vi "util-path.vi"(6 "Create Folders?(F)":bool, 8 "error in":errorcluster, 10 "Selected Folder (PROCS)":T1, 11 "append path (ie. folder\\filename.*)":string) -> (0 "error out":errorcluster, 1 "SelectedPath Filenames":string[](array[string]), 2 "SelectedPath":path, 3 "AppPath":path, 4 ".extension (.prc)":string)   [LabVIEW 2024]
uses:
  controls/typePathSelector.ctl
panel:
  # "path to file:  folder1\\...\\filename.*"
  # "build path example:\n\nAppend to may be a path to folder (123\\456) or a path to file (123\\456.*)\n\nif specific folder is selected (Procedures, templates, logs etc.) the code tries \nto add a file extansion by replacing *. in the provided path (Append To)\n\nif there is no filename (hence no .* at the end) the path in Append To considered \npath to folder.\n\nAppend To examples: \n\"123\\456\" a path to folder\n\"123\\456.*\" a path to file (.* will be replaced either by empty string or selected folder's extansion)"
  # "Append folder to result paths"
  # "Select a folder to output as Selected Folder"
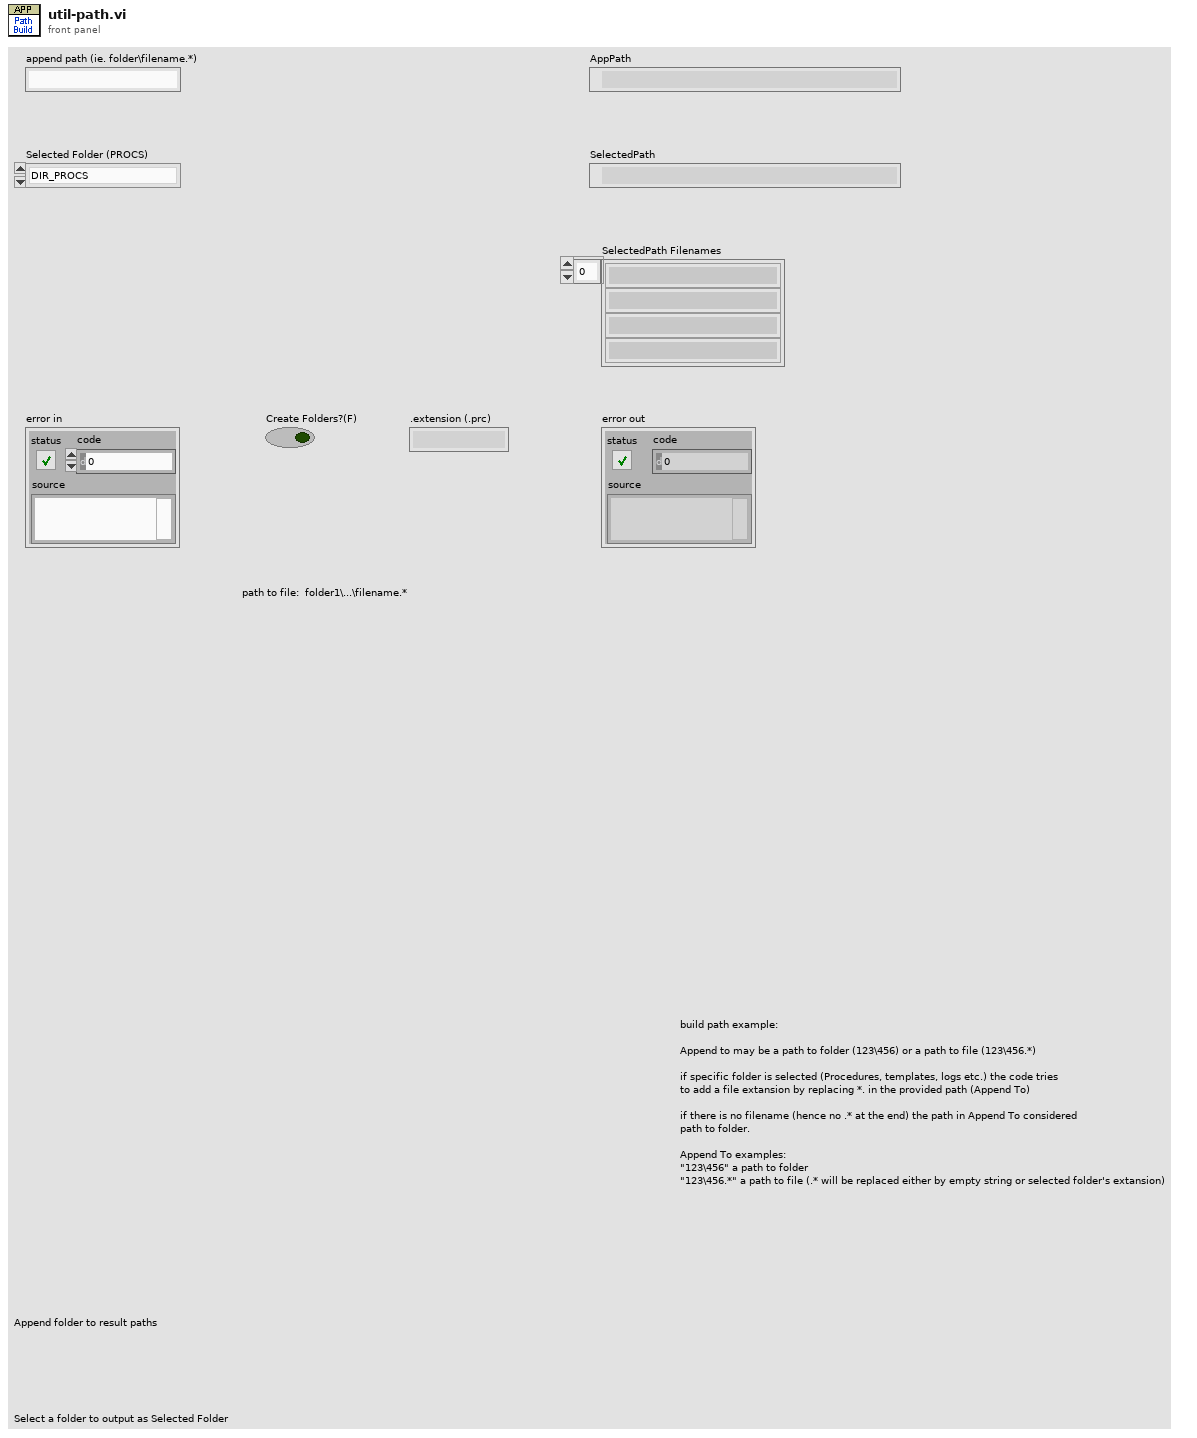
[diagram p1: front panel]
types:
  T1 = typedef "typePathSelector.ctl" = enum16{"DIR_PROCS", "DIR_CONFIG", "DIR_TEMPLATE", "DIR_IO_FILE", "DIR_RECORD", "DIR_LOG", "DIR_RUNTIME", "DIR_PRESET", "DIR_INI"}
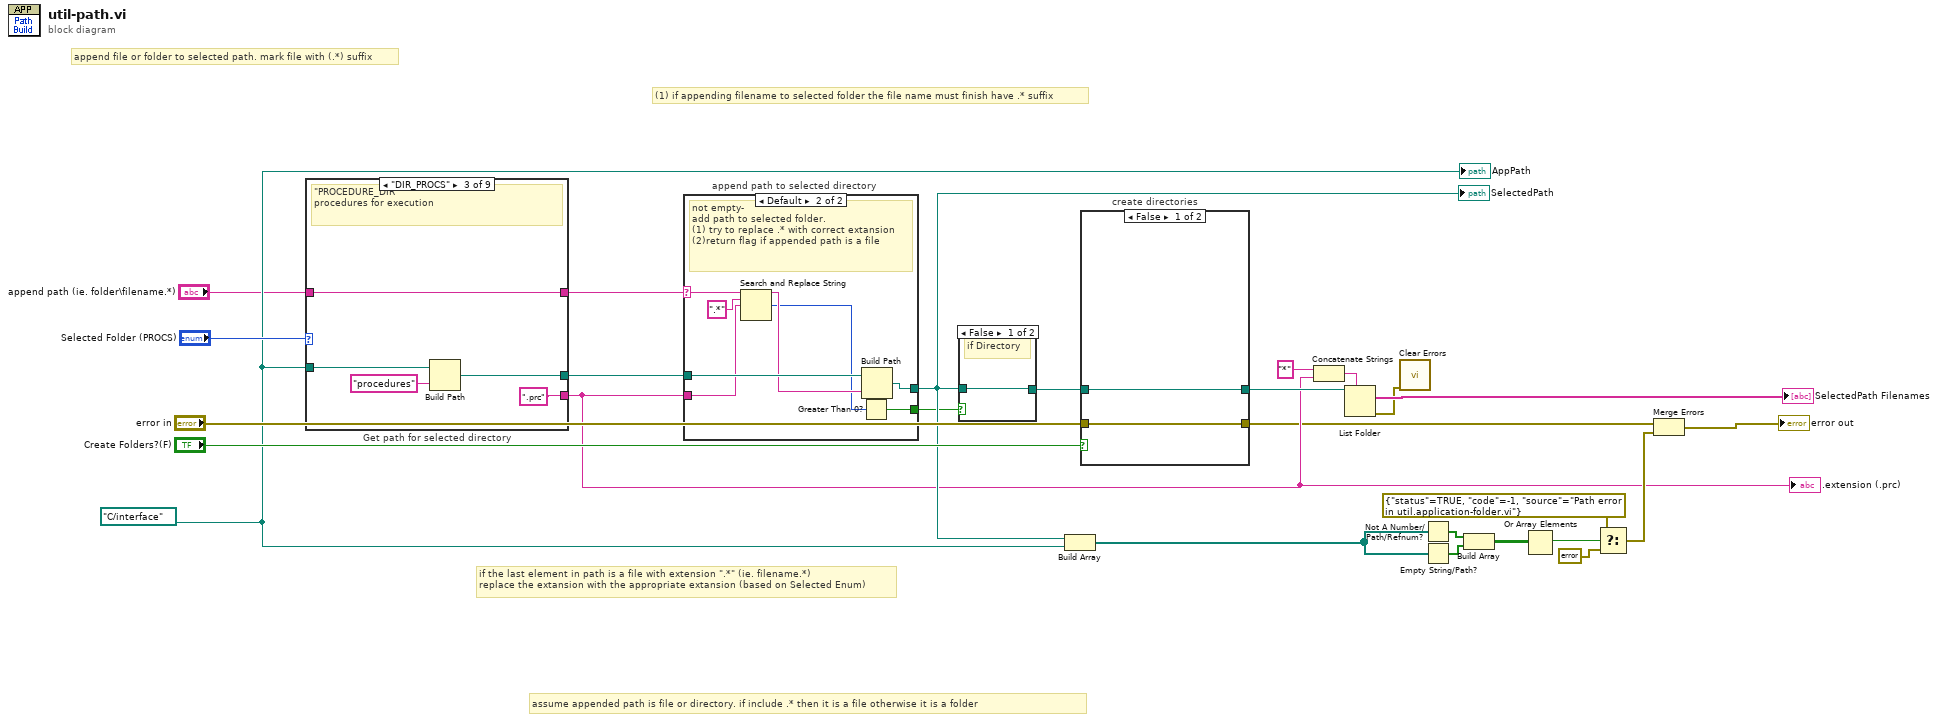
[diagram p0: block diagram]
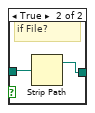
[diagram p2: hidden frame]
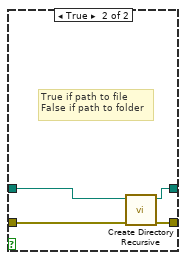
[diagram p3: hidden frame]
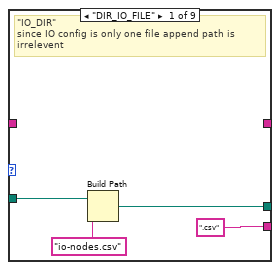
[diagram p5: hidden frame]
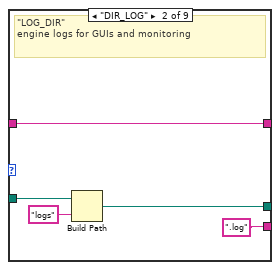
[diagram p6: hidden frame]
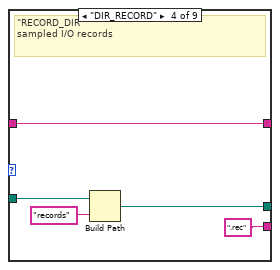
[diagram p7: hidden frame]
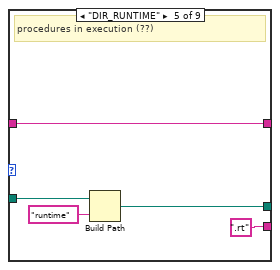
[diagram p8: hidden frame]
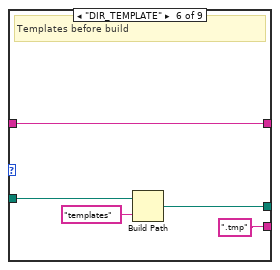
[diagram p9: hidden frame]
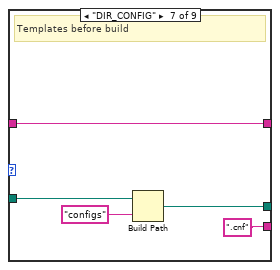
[diagram p10: hidden frame]
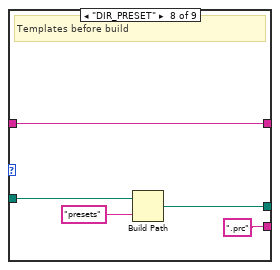
[diagram p11: hidden frame]
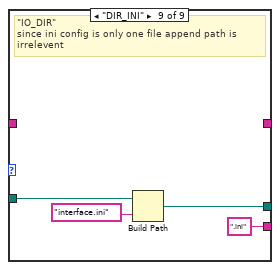
[diagram p12: hidden frame]
diagram:
  w7 = path "C:/interface" ("file path (use dialog)")
  # "assume appended path is file or directory. if include .* then it is a file otherwise it is a folder"
  # "(1) if appending filename to selected folder the file name must finish have .* suffix"
  # "if the last element in path is a file with extension \".*\" (ie. filename.*)\nreplace the extansion with the appropriate extansion (based on Selected Enum)"
  # "append file or folder to selected path. mark file with (.*) suffix"
  n1 = case "Get path for selected directory" shown="\"DIR_PROCS\"" "Selected Folder (PROCS)" {
    tunnel: [w28 w33 w38 w43 w48 w53 w58 w63 w67] -> w23
    tunnel: w7 -> [w30 w35 w40 w45 w50 w55 w60 w65 w69]
    tunnel: [".csv" ("pattern") ".log" ("pattern") ".prc" ("pattern") ".rec" ("pattern") ".rt" ("pattern") ".tmp" ("pattern") ".cnf" ("pattern") ".prc" ("pattern") ".ini" ("pattern")] -> w10
    tunnel: "append path (ie. folder\\filename.*)" -> [_ w31 w36 w41 w46 w51 w56 w61 _]
    tunnel: [_ w31 w36 w41 w46 w51 w56 w61 _] -> w1
    frame "DIR_IO_FILE" {
      # "\"IO_DIR\"\nsince IO config is only one file append path is irrelevent"
      n2 = Build Path(base path=w30, name or relative path="io-nodes.csv") -> (appended path=w28:path)
    }
    frame "DIR_LOG" {
      # "\"LOG_DIR\" \nengine logs for GUIs and monitoring"
      n3 = Build Path(base path=w35, name or relative path="logs") -> (appended path=w33:path)
    }
    frame "DIR_PROCS" {
      # "\"PROCEDURE_DIR\" \nprocedures for execution"
      n4 = Build Path(base path=w40, name or relative path="procedures") -> (appended path=w38:path)
    }
    frame "DIR_RECORD" {
      # "\"RECORD_DIR\" \nsampled I/O records"
      n5 = Build Path(base path=w45, name or relative path="records") -> (appended path=w43:path)
    }
    frame "DIR_RUNTIME" {
      # "procedures in execution (??)"
      n6 = Build Path(base path=w50, name or relative path="runtime") -> (appended path=w48:path)
    }
    frame "DIR_TEMPLATE" {
      # "Templates before build"
      n7 = Build Path(base path=w55, name or relative path="templates") -> (appended path=w53:path)
    }
    frame "DIR_CONFIG" {
      # "Templates before build"
      n8 = Build Path(base path=w60, name or relative path="configs") -> (appended path=w58:path)
    }
    frame "DIR_PRESET" {
      # "Templates before build"
      n9 = Build Path(base path=w65, name or relative path="presets") -> (appended path=w63:path)
    }
    frame "DIR_INI" {
      # "\"IO_DIR\"\nsince ini config is only one file append path is irrelevent"
      n10 = Build Path(base path=w69, name or relative path="interface.ini") -> (appended path=w67:path)
    }
  }
  ".extension (.prc)" <- w10
  n11 = case "append path to selected directory" shown="Default" w1 {
    selector: w1 -> [_ w72]
    tunnel: [w70 w78] -> w11
    tunnel: w23 -> [w70 w77]
    tunnel: w10 -> [_ w71]
    tunnel: [_ w73] -> w3
    frame "" {
      # "empty\nDON'T append to selected folder"
    }
    frame Default {
      # "not empty- \nadd path to selected folder.\n(1) try to replace .* with correct extansion\n(2)return flag if appended path is a file"
      n12 = Search and Replace String(input string=w72, search string=".*", replace string=w71) -> (result string=w76:string, number of replacements=w74:i32)  [unwired: 5 in, 2 out]
      n13 = Greater Than 0?(x=w74) -> (x > 0?=w73:bool)
      n14 = Build Path(base path=w77, name or relative path=w76) -> (appended path=w78:path)
    }
  }
  "SelectedPath" <- w11
  n15 = case shown="False" w3 {
    tunnel: w11 -> [w79 w80]
    tunnel: [w79 w81] -> w6
    frame False {
      # "if Directory"
    }
    frame True {
      # "if File?"
      n16 = Strip Path(path=w80) -> (stripped path=w81:path)  [unwired: 1 out]
    }
  }
  n17 = Build Array(w11, w7) -> (w20:path[])
  n18 = case "create directories" shown="False" "Create Folders?(F)" {
    tunnel: [w83 w87] -> w5
    tunnel: "error in" -> [w83 w86]
    tunnel: [w82 w85] -> w22
    tunnel: w6 -> [w82 w84]
    frame False {
    }
    frame True {
      # "True if path to file\nFalse if path to folder"
      n19 = call <vilib>:"Create Directory Recursive.vi"("error in (no error)"=w86, "directory"=w84) -> ("error out"=w87:errorcluster, "directory copy"=w85:path)  [unwired: 3 in, 1 out]
    }
  }
  n20 = Concatenate Strings("*" ("pattern"), w10) -> (w8:string)
  n21 = List Folder(path=w22, pattern=w8) -> (filenames=→"SelectedPath Filenames":string[], error out=w4:errorcluster)  [unwired: 2 in, 2 out]
  n22 = call <vilib>:"Clear Errors.vi"("error in (no error)"=w4) -> ()  [unwired: 5 in, 2 out]
  n23 = Not A Number/Path/Refnum?(number/path/refnum=w20) -> (NaN/Path/Refnum?=w19:bool[])
  n24 = Empty String/Path?(string/path=w20) -> (empty?=w18:bool[])
  n25 = Build Array(w19, w18) -> (w17:bool[][])
  n26 = Or Array Elements(Boolean array=w17) -> (logical OR=w16:bool)
  n27 = Select(t=errorcluster {"status"=TRUE, "code"=-1, "source"="Path error in util.application-folder.vi"} ("error out"), s=w16, f=errorcluster {"status"=FALSE, "code"=0, "source"=""}) -> (s? t:f=w13:errorcluster)
  n28 = Merge Errors(w5, w13) -> (→"error out":errorcluster)
  "AppPath" <- w7
